vi "Do Result.vi"(5 "Round":u32, 6 "Teams in":refnum<class "Team.lvclass">[](array[class]), 7 "Position":T1, 8 "Run Result":T2, 9 "Square":refnum<class "Square.lvclass">, 10 "Team":i32, 11 "Map in":refnum<class "Map.lvclass">) -> (3 "Map out":refnum<class "Map.lvclass">, 4 "Teams out":refnum<class "Team.lvclass">[](array[class]))   [LabVIEW 2020, in "SquareBattle.lvlib" / "Map.lvclass"]
uses:
  Map.lvclass
  Map.lvclass/Map.ctl
  Action.ctl
  SquareBattle.lvlib
  Square/Square.lvclass
  Direction.ctl
  Run Result.ctl
  Position.ctl
  Team/Team.lvclass
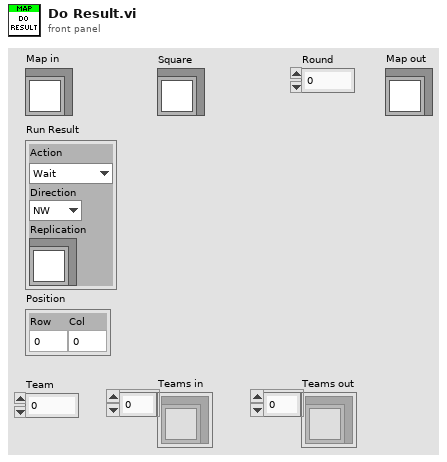
[diagram p1: front panel]
types:
  T1 = typedef "SquareBattle.lvlib/Position.ctl" = cluster{"Row":i32, "Col":i32}
  T2 = typedef "SquareBattle.lvlib/Run Result.ctl" = cluster{"Action":T3, "Direction":T4, "Replication":refnum<class "Square.lvclass">}
  T3 = typedef "SquareBattle.lvlib/Action.ctl" = enum16{"Wait", "Move", "Attack", "Replicate"}
  T4 = typedef "SquareBattle.lvlib/Direction.ctl" = enum16{"NW", "N", "NE", "E", "SE", "S", "SW", "W"}
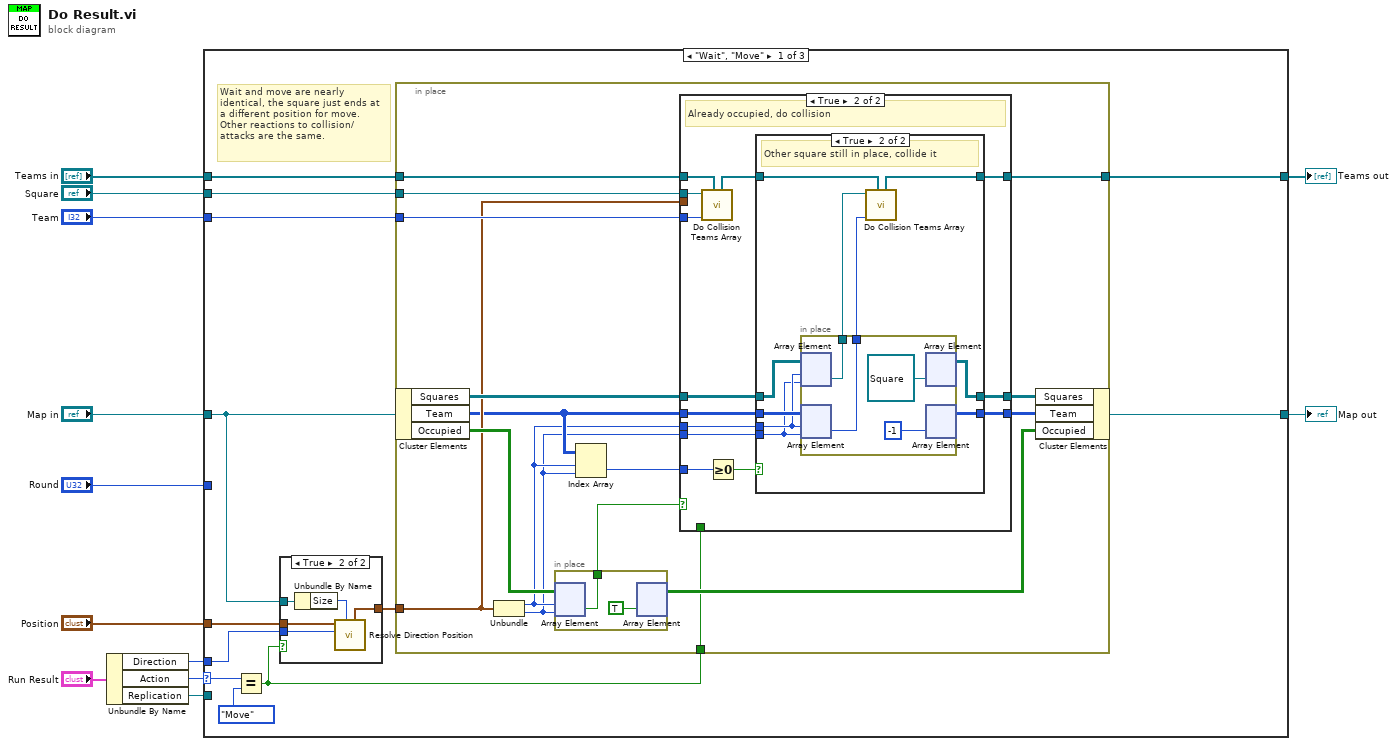
[diagram p0: block diagram]
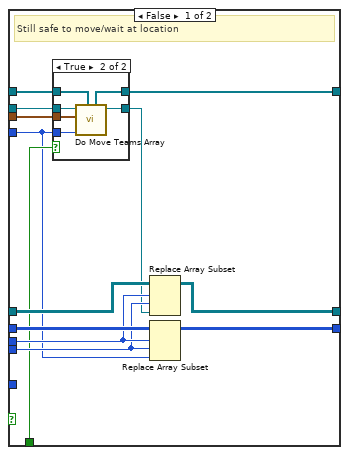
[diagram p3: hidden frame]
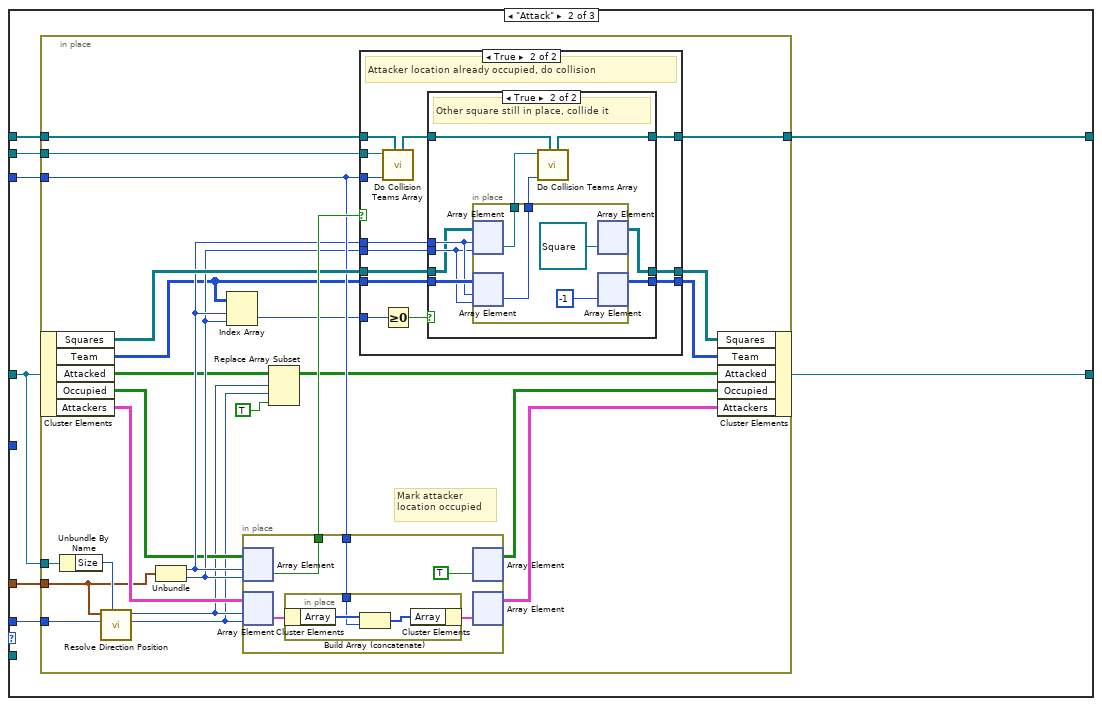
[diagram p6: hidden frame]
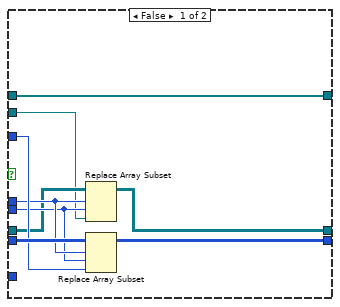
[diagram p7: hidden frame]
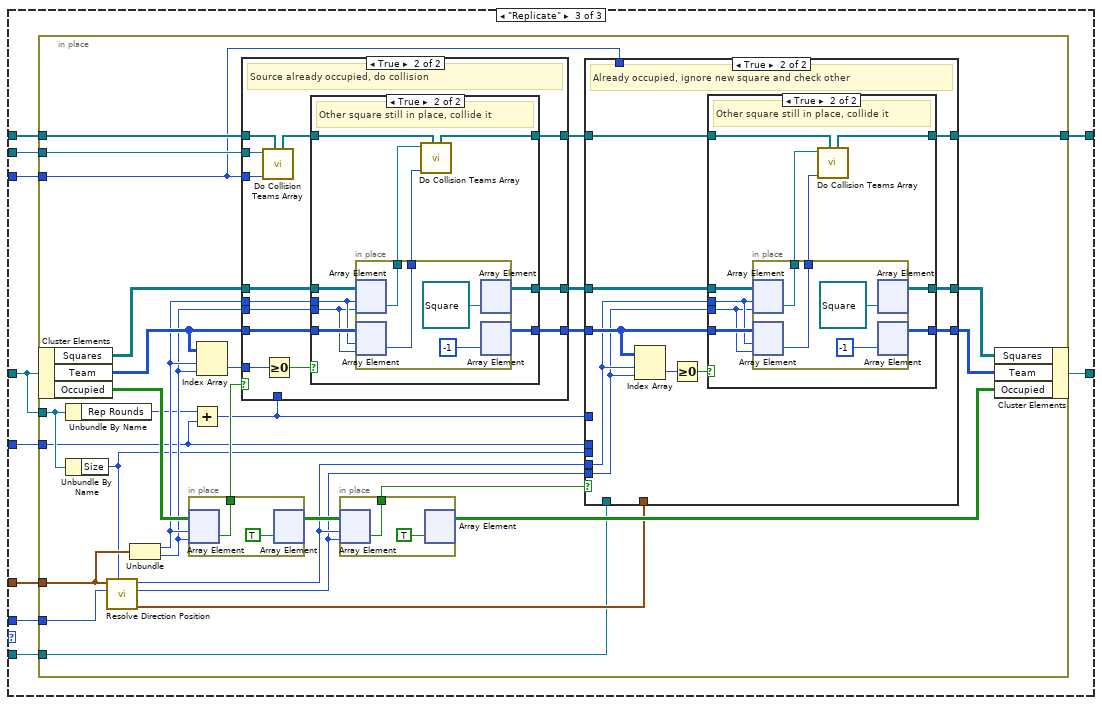
[diagram p9: hidden frame]
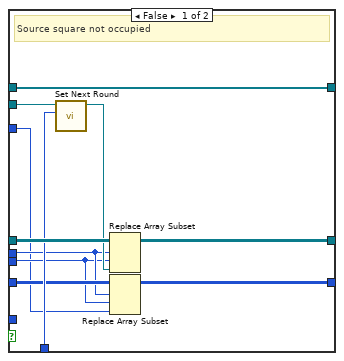
[diagram p10: hidden frame]
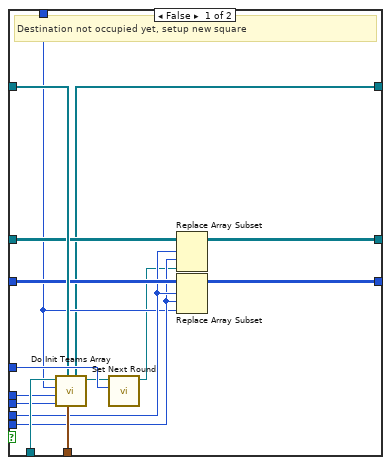
[diagram p12: hidden frame]
diagram:
  n1 = Unbundle By Name("Run Result") -> ("Direction"=w11:T4, "Action"=w9:T3, "Replication"=w8:refnum<class "Square.lvclass">)
  n2 = case shown="\"Wait\", \"Move\"" w9 {
    selector: w9 -> [w16 _ _]
    tunnel: "Position" -> [w19 w107 w187]
    tunnel: w8 -> [_ _ w188]
    tunnel: "Team" -> [w23 w103 w186]
    tunnel: "Square" -> [w24 w102 w185]
    tunnel: "Map in" -> [w17 w106 w183]
    tunnel: "Teams in" -> [w22 w101 w184]
    tunnel: [w21 w100 w180] -> w3
    tunnel: [w20 w104 w182] -> w2
    tunnel: w11 -> [w14 w105 w189]
    tunnel: "Round" -> [_ _ w181]
    frame "Wait", "Move" {
      # "Wait and move are nearly identical, the square just ends at a different position for move. Other reactions to collision/attacks are the same."
      n3 = Equal?(x=w16, y=Action."Move") -> (x = y?=w13:bool)
      n4 = case shown="True" w13 {
        tunnel: w19 -> [w25 w30]
        tunnel: [w25 w28] -> w18
        tunnel: w17 -> [_ w27]
        tunnel: w14 -> [_ w29]
        frame False {
        }
        frame True {
          n5 = Unbundle By Name(w27) -> ("Size"=w26:i32)
          n6 = call "Resolve Direction Position.vi"("Board Size"=w26, "Direction"=w29, "From"=w30) -> ("To"=w28:T1)  [unwired: 6 in, 2 out]
        }
      }
      n7 = in-place {
        in-place-border: w24 -> [w43]
        in-place-border: w18 -> [w36]
        in-place-border: w23 -> [w42]
        in-place-border: w22 -> [w39]
        in-place-border: [w38] -> w21
        in-place-border: w13 -> [w37]
        n8 = in-place-cluster #1(w17) -> ("Squares"=w44:refnum<class "Square.lvclass">[][], "Team"=w34:i32[][], "Occupied"=w46:bool[][])
        n9 = Unbundle(w36) -> ("Row"=w33:i32, "Col"=w32:i32)
        n10 = in-place {
          in-place-border: [w98] -> w35
          n11 = in-place-array #2(w46, w33, w32) -> (w98:bool)
          n12 = in-place-array #2(TRUE ("element")) -> (w45:bool[][])  [unwired: 2 out]
        }
        n13 = Index Array(array=w34, index (row)=w33, index (col)=w32) -> (element=w31:i32)
        n14 = case shown="True" w35 {
          tunnel: w44 -> [w58 w75]
          tunnel: w34 -> [w59 w77]
          tunnel: w43 -> [w51 w80]
          tunnel: w33 -> [w57 w74]
          tunnel: w32 -> [w56 w73]
          tunnel: w42 -> [w47 w78]
          tunnel: [w55 w76] -> w41
          tunnel: [w54 w70] -> w40
          tunnel: w39 -> [w53 w79]
          tunnel: [w50 w72] -> w38
          tunnel: w37 -> [w52 _]
          tunnel: w36 -> [w49 _]
          tunnel: w31 -> [_ w69]
          frame False {
            # "Still safe to move/wait at location"
            n15 = case shown="True" w52 {
              tunnel: w53 -> [w60 w67]
              tunnel: w51 -> [w61 w65]
              tunnel: [w60 w66] -> w50
              tunnel: [w61 w63] -> w48
              tunnel: w49 -> [_ w64]
              tunnel: w47 -> [_ w62]
              frame False {
              }
              frame True {
                n16 = call "Do Move Teams Array.vi"("Teams in"=w67, "Team"=w62, "Position"=w64, "Square in"=w65) -> ("Square out"=w63:refnum<class "Square.lvclass">, "Teams out"=w66:refnum<class "Team.lvclass">[])  [unwired: 6 in]
              }
            }
            n17 = Replace Array Subset(array=w58, new element=w48, index (row)=w57, index (col)=w56) -> (w54:refnum<class "Square.lvclass">[][])
            n18 = Replace Array Subset(array=w59, new element=w47, index (row)=w57, index (col)=w56) -> (w55:i32[][])
          }
          frame True {
            # "Already occupied, do collision"
            n19 = call "Do Collision Teams Array.vi"("Teams In"=w79, "Team"=w78, "Square"=w80) -> ("Teams out"=w71:refnum<class "Team.lvclass">[])  [unwired: 8 in]
            n20 = Greater Or Equal To 0?(x=w69) -> (x >= 0?=w68:bool)
            n21 = case shown="True" w68 {
              tunnel: w75 -> [w82 w92]
              tunnel: w77 -> [w81 w93]
              tunnel: w71 -> [w83 w89]
              tunnel: [w83 w88] -> w72
              tunnel: [w82 w86] -> w70
              tunnel: [w81 w87] -> w76
              tunnel: w74 -> [_ w85]
              tunnel: w73 -> [_ w84]
              frame False {
              }
              frame True {
                # "Other square still in place, collide it"
                n22 = in-place {
                  in-place-border: [w96] -> w90
                  in-place-border: [w95] -> w91
                  n23 = in-place-array #3(w92, w85, w84) -> (w95:refnum<class "Square.lvclass">)
                  n24 = in-place-array #4(w93, w85, w84) -> (w96:i32)
                  n25 = in-place-array #3(refnum<class "Square.lvclass"> refnum ("element")) -> (w86:refnum<class "Square.lvclass">[][])  [unwired: 2 out]
                  n26 = in-place-array #4(-1 ("element")) -> (w87:i32[][])  [unwired: 2 out]
                }
                n27 = call "Do Collision Teams Array.vi"("Teams In"=w89, "Team"=w90, "Square"=w91) -> ("Teams out"=w88:refnum<class "Team.lvclass">[])  [unwired: 8 in]
              }
            }
          }
        }
        n28 = in-place-cluster #1("Squares"=w40, "Team"=w41, "Occupied"=w45) -> (w20:refnum<class "Map.lvclass">)
      }
    }
    frame "Attack" {
      n29 = in-place {
        in-place-border: w107 -> [w123]
        in-place-border: w106 -> [w131]
        in-place-border: w105 -> [w129]
        in-place-border: w103 -> [w126]
        in-place-border: w102 -> [w125]
        in-place-border: w101 -> [w124]
        in-place-border: [w108] -> w100
        # "Mark attacker location occupied"
        n30 = in-place-cluster #5(w106) -> ("Squares"=w127:refnum<class "Square.lvclass">[][], "Team"=w118:i32[][], "Attacked"=w116:bool[][], "Occupied"=w117:bool[][], "Attackers"=w132:cluster{"Array":i32[]}[][])
        n31 = Unbundle By Name(w131) -> ("Size"=w130:i32)
        n32 = call "Resolve Direction Position.vi"("Board Size"=w130, "Direction"=w129, "From"=w123) -> ("Col"=w114:i32, "Row"=w115:i32)  [unwired: 6 in, 1 out]
        n33 = Unbundle(w123) -> ("Row"=w121:i32, "Col"=w120:i32)
        n34 = Index Array(array=w118, index (row)=w121, index (col)=w120) -> (element=w119:i32)
        n35 = in-place {
          in-place-border: w126 -> [w174]
          in-place-border: [w172] -> w128
          n36 = in-place-array #6(w117, w121, w120) -> (w172:bool)
          n37 = in-place-array #7(w132, w115, w114) -> (w176:cluster{"Array":i32[]})
          n38 = in-place {
            in-place-border: w174 -> [w178]
            n39 = in-place-cluster #8(w176) -> ("Array"=w179:i32[])
            n40 = Build Array (concatenate)(w179, w178) -> (w177:i32[])
            n41 = in-place-cluster #8("Array"=w177) -> (w175:cluster{"Array":i32[]})
          }
          n42 = in-place-array #6(TRUE ("element")) -> (w112:bool[][])  [unwired: 2 out]
          n43 = in-place-array #7(w175) -> (w122:cluster{"Array":i32[]}[][])  [unwired: 2 out]
        }
        n44 = Replace Array Subset(array=w116, new element=TRUE ("new element/subarray"), index (row)=w115, index (col)=w114) -> (w111:bool[][])
        n45 = case shown="True" w128 {
          tunnel: [w136 w145] -> w109
          tunnel: [w139 w144] -> w110
          tunnel: w121 -> [w138 w150]
          tunnel: w120 -> [w137 w149]
          tunnel: w126 -> [w140 w154]
          tunnel: w125 -> [w133 w153]
          tunnel: w124 -> [w135 w152]
          tunnel: [w135 w151] -> w108
          tunnel: w119 -> [_ w148]
          tunnel: w127 -> [w134 w147]
          tunnel: w118 -> [w141 w146]
          frame False {
            n46 = Replace Array Subset(array=w134, new element=w133, index (row)=w138, index (col)=w137) -> (w136:refnum<class "Square.lvclass">[][])
            n47 = Replace Array Subset(array=w141, new element=w140, index (row)=w138, index (col)=w137) -> (w139:i32[][])
          }
          frame True {
            # "Attacker location already occupied, do collision"
            n48 = call "Do Collision Teams Array.vi"("Teams In"=w152, "Team"=w154, "Square"=w153) -> ("Teams out"=w142:refnum<class "Team.lvclass">[])  [unwired: 8 in]
            n49 = Greater Or Equal To 0?(x=w148) -> (x >= 0?=w143:bool)
            n50 = case shown="True" w143 {
              tunnel: w147 -> [w156 w164]
              tunnel: w146 -> [w155 w167]
              tunnel: w142 -> [w157 w161]
              tunnel: [w157 w160] -> w151
              tunnel: w150 -> [_ w166]
              tunnel: w149 -> [_ w165]
              tunnel: [w156 w158] -> w145
              tunnel: [w155 w159] -> w144
              frame False {
              }
              frame True {
                # "Other square still in place, collide it"
                n51 = in-place {
                  in-place-border: [w170] -> w162
                  in-place-border: [w169] -> w163
                  n52 = in-place-array #9(w164, w166, w165) -> (w169:refnum<class "Square.lvclass">)
                  n53 = in-place-array #10(w167, w166, w165) -> (w170:i32)
                  n54 = in-place-array #9(refnum<class "Square.lvclass"> refnum ("element")) -> (w158:refnum<class "Square.lvclass">[][])  [unwired: 2 out]
                  n55 = in-place-array #10(-1 ("element")) -> (w159:i32[][])  [unwired: 2 out]
                }
                n56 = call "Do Collision Teams Array.vi"("Teams In"=w161, "Team"=w162, "Square"=w163) -> ("Teams out"=w160:refnum<class "Team.lvclass">[])  [unwired: 8 in]
              }
            }
          }
        }
        n57 = in-place-cluster #5("Squares"=w109, "Team"=w110, "Attacked"=w111, "Occupied"=w112, "Attackers"=w122) -> (w104:refnum<class "Map.lvclass">)
      }
    }
    frame "Replicate" {
      n58 = in-place {
        in-place-border: w189 -> [w219]
        in-place-border: w188 -> [w193]
        in-place-border: w187 -> [w217]
        in-place-border: w186 -> [w201]
        in-place-border: w185 -> [w210]
        in-place-border: w184 -> [w209]
        in-place-border: w183 -> [w218]
        in-place-border: w181 -> [w196]
        in-place-border: [w190] -> w180
        n59 = in-place-cluster #11(w183) -> ("Squares"=w212:refnum<class "Square.lvclass">[][], "Team"=w207:i32[][], "Occupied"=w216:bool[][])
        n60 = Unbundle By Name(w218) -> ("Rep Rounds"=w198:u32)
        n61 = Unbundle By Name(w218) -> ("Size"=w194:i32)
        n62 = call "Resolve Direction Position.vi"("Board Size"=w194, "Direction"=w219, "From"=w217) -> ("Col"=w199:i32, "Row"=w200:i32, "To"=w195:T1)  [unwired: 6 in]
        n63 = Unbundle(w217) -> ("Row"=w203:i32, "Col"=w202:i32)
        n64 = in-place {
          in-place-border: [w307] -> w211
          n65 = in-place-array #12(w216, w203, w202) -> (w307:bool)
          n66 = in-place-array #12(TRUE ("element")) -> (w215:bool[][])  [unwired: 2 out]
        }
        n67 = Add(x=w198, y=w196) -> (x+y=w197:u32)
        n68 = Index Array(array=w207, index (row)=w203, index (col)=w202) -> (element=w206:i32)
        n69 = case shown="True" w211 {
          tunnel: w212 -> [w229 w235]
          tunnel: w207 -> [w224 w236]
          tunnel: w201 -> [w221 w241]
          tunnel: w210 -> [w228 w243]
          tunnel: w209 -> [w230 w242]
          tunnel: [w230 w240] -> w208
          tunnel: w206 -> [_ w238]
          tunnel: [w226 w234] -> w205
          tunnel: [w220 w233] -> w204
          tunnel: w203 -> [w223 w232]
          tunnel: w202 -> [w222 w231]
          tunnel: w197 -> [w227 _]
          frame False {
            # "Source square not occupied"
            n70 = call "Set Next Round.vi"("Next Round"=w227, "Square in"=w228) -> ("Square out"=w225:refnum<class "Square.lvclass">)  [unwired: 9 in]
            n71 = Replace Array Subset(array=w229, new element=w225, index (row)=w223, index (col)=w222) -> (w226:refnum<class "Square.lvclass">[][])
            n72 = Replace Array Subset(array=w224, new element=w221, index (row)=w223, index (col)=w222) -> (w220:i32[][])
          }
          frame True {
            # "Source already occupied, do collision"
            n73 = call "Do Collision Teams Array.vi"("Teams In"=w242, "Team"=w241, "Square"=w243) -> ("Teams out"=w239:refnum<class "Team.lvclass">[])  [unwired: 8 in]
            n74 = Greater Or Equal To 0?(x=w238) -> (x >= 0?=w237:bool)
            n75 = case shown="True" w237 {
              tunnel: w235 -> [w245 w253]
              tunnel: w236 -> [w244 w256]
              tunnel: w239 -> [w246 w250]
              tunnel: [w246 w249] -> w240
              tunnel: w232 -> [_ w255]
              tunnel: w231 -> [_ w254]
              tunnel: [w245 w247] -> w234
              tunnel: [w244 w248] -> w233
              frame False {
              }
              frame True {
                # "Other square still in place, collide it"
                n76 = in-place {
                  in-place-border: [w259] -> w251
                  in-place-border: [w258] -> w252
                  n77 = in-place-array #13(w253, w255, w254) -> (w258:refnum<class "Square.lvclass">)
                  n78 = in-place-array #14(w256, w255, w254) -> (w259:i32)
                  n79 = in-place-array #13(refnum<class "Square.lvclass"> refnum ("element")) -> (w247:refnum<class "Square.lvclass">[][])  [unwired: 2 out]
                  n80 = in-place-array #14(-1 ("element")) -> (w248:i32[][])  [unwired: 2 out]
                }
                n81 = call "Do Collision Teams Array.vi"("Teams In"=w250, "Team"=w251, "Square"=w252) -> ("Teams out"=w249:refnum<class "Team.lvclass">[])  [unwired: 8 in]
              }
            }
          }
        }
        n82 = in-place {
          in-place-border: [w305] -> w213
          n83 = in-place-array #15(w215, w200, w199) -> (w305:bool)
          n84 = in-place-array #15(TRUE ("element")) -> (w214:bool[][])  [unwired: 2 out]
        }
        n85 = case shown="True" w213 {
          tunnel: w208 -> [w273 w285]
          tunnel: w193 -> [w274 _]
          tunnel: w205 -> [w270 w286]
          tunnel: w204 -> [w269 w283]
          tunnel: w201 -> [w265 _]
          tunnel: w200 -> [w267 w282]
          tunnel: w199 -> [w266 w281]
          tunnel: w197 -> [w276 _]
          tunnel: w196 -> [w268 _]
          tunnel: w195 -> [w275 _]
          tunnel: w194 -> [w271 _]
          tunnel: [w263 w277] -> w192
          tunnel: [w262 w278] -> w191
          tunnel: [w261 w284] -> w190
          frame False {
            # "Destination not occupied yet, setup new square"
            n86 = call "Do Init Teams Array.vi"("Position"=w275, "Teams in"=w273, "Board Size"=w271, "Round"=w268, "Team"=w265, "Square in"=w274) -> ("Square out"=w272:refnum<class "Square.lvclass">, "Teams out"=w261:refnum<class "Team.lvclass">[])  [unwired: 4 in]
            n87 = call "Set Next Round.vi"("Next Round"=w276, "Square in"=w272) -> ("Square out"=w264:refnum<class "Square.lvclass">)  [unwired: 9 in]
            n88 = Replace Array Subset(array=w270, new element=w264, index (row)=w267, index (col)=w266) -> (w262:refnum<class "Square.lvclass">[][])
            n89 = Replace Array Subset(array=w269, new element=w265, index (row)=w267, index (col)=w266) -> (w263:i32[][])
          }
          frame True {
            # "Already occupied, ignore new square and check other"
            n90 = Index Array(array=w283, index (row)=w282, index (col)=w281) -> (element=w280:i32)
            n91 = Greater Or Equal To 0?(x=w280) -> (x >= 0?=w279:bool)
            n92 = case shown="True" w279 {
              tunnel: w286 -> [w288 w296]
              tunnel: w283 -> [w287 w299]
              tunnel: w285 -> [w289 w293]
              tunnel: [w289 w292] -> w284
              tunnel: w282 -> [_ w298]
              tunnel: w281 -> [_ w297]
              tunnel: [w288 w290] -> w278
              tunnel: [w287 w291] -> w277
              frame False {
              }
              frame True {
                # "Other square still in place, collide it"
                n93 = in-place {
                  in-place-border: [w302] -> w294
                  in-place-border: [w301] -> w295
                  n94 = in-place-array #16(w296, w298, w297) -> (w301:refnum<class "Square.lvclass">)
                  n95 = in-place-array #17(w299, w298, w297) -> (w302:i32)
                  n96 = in-place-array #16(refnum<class "Square.lvclass"> refnum ("element")) -> (w290:refnum<class "Square.lvclass">[][])  [unwired: 2 out]
                  n97 = in-place-array #17(-1 ("element")) -> (w291:i32[][])  [unwired: 2 out]
                }
                n98 = call "Do Collision Teams Array.vi"("Teams In"=w293, "Team"=w294, "Square"=w295) -> ("Teams out"=w292:refnum<class "Team.lvclass">[])  [unwired: 8 in]
              }
            }
          }
        }
        n99 = in-place-cluster #11("Squares"=w191, "Team"=w192, "Occupied"=w214) -> (w182:refnum<class "Map.lvclass">)
      }
    }
  }
  "Map out" <- w2
  "Teams out" <- w3
